vi "Write Tx Data (CDB WDT).vi"(0 "Register Bus":T1, 5 "data":waveform(cdb), 9 "timeout (s)":dbl=10.0, 11 "error in":errorcluster) -> (4 "Register Bus (out)":T1, 15 "error out":errorcluster)   [LabVIEW 2017]
doc: "Write Tx data to the device. It's required to call <b>Configure Stream</b> and <b>Initiate Stream</b> before calling this VI.\n\n<B>Input Parameters</B>\n\n<B>Register Bus</B> The Register Bus object created by the ni579x Open VI and used as the session handle for the NI-579x Configuration Design Library.\n\n<B>data</B> is the Tx data to write to the device.\n\n<B>timeout (s)</B> is how long to wait for (in seconds).\n\n<B>error in</B> describes error conditions that occur before this node runs. This input provides standard 'error in' functionality.\n\n<B>Output Parameters</B>\n\n<B>Register Bus (out)</B> The Register Bus object created by the ni579x Open VI and used as the session handle for the NI-579x Configuration Design Library.\n\n<B>error out</B> contains error information. This output provides standard 'error out' functionality."
uses:
  <instrlib>/_niInstr/Register Bus/v0/Host/Public/Register Bus Session.ctl
  <instrlib>/_niInstr/Register Bus/v0/Host/Private/Session Data.ctl
  Tx FPGA VI Reference.ctl
  <vilib>/Utility/error.llb/Error Cluster From Error Code.vi
  <vilib>/rvi/errors/niLvFpgaAdjustHostInterfaceError.vi
  <vilib>/rvi/interface/nirviMethod/nirviMethod.xnode
  <instrlib>/_niInstr/Register Bus/v0/Host/niInstr Register Bus v0 Host.lvlib
  <vilib>/FPGAPlugInAG/Dynamic/niLvFpga_WriteFifo_Dynamic.vi
  <vilib>/rvi/errors/niLvFpgaMergeErrorWithErrorCode.vi
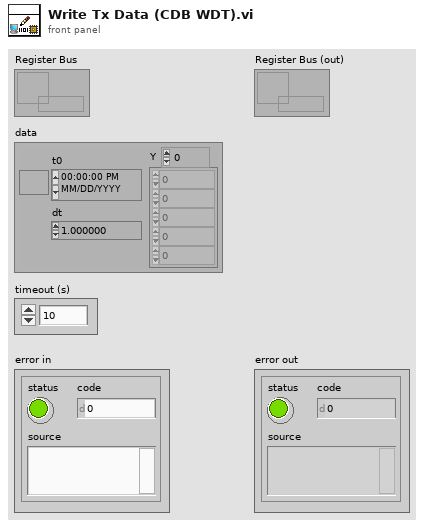
[diagram p1: front panel]
types:
  T1 = typedef "niInstr Register Bus v0 Host.lvlib/Register Bus Session.ctl" = refnum<queue>
  T2 = typedef "Tx FPGA VI Reference.ctl" = refnum<k20>
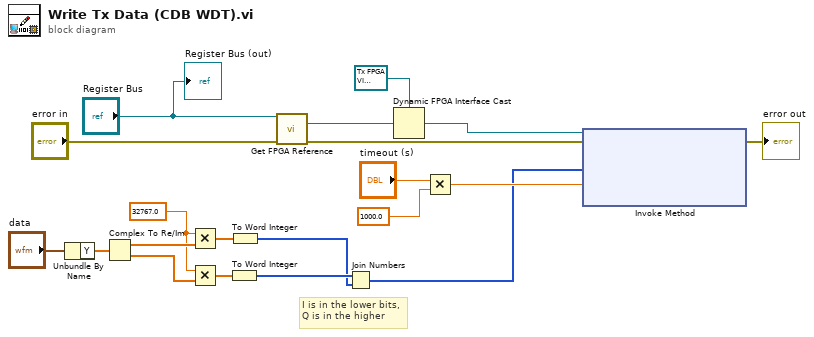
[diagram p0: block diagram]
diagram:
  w5 = 32767.0
  # "I is in the lower bits,\nQ is in the higher"
  n1 = Unbundle By Name("data") -> ("Y"=w8:cdb[])
  n2 = Complex To Re/Im(x + iy=w8) -> (x=w7:dbl[], y=w6:dbl[])
  n3 = Multiply(x=w5, y=w7) -> (x*y=w4:dbl[])
  n4 = Multiply(x=w5, y=w6) -> (x*y=w3:dbl[])
  n5 = To Word Integer(number=w3) -> (16bit integer=w2:i16[])
  n6 = To Word Integer(number=w4) -> (16bit integer=w1:i16[])
  n7 = call <instrlib>:"Get FPGA Reference.vi"("session in"="Register Bus", "error in"="error in") -> ("fpga ref"=w17:refnum<k20>, "error out"=w11:errorcluster)  [unwired: 11 in, 1 out]
  n8 = Join Numbers(hi=w2, lo=w1) -> ((hi.lo)=w10:u32[])
  n9 = Dynamic FPGA Interface Cast(Session In=T2 refnum ("Type"), Type=w17) -> (Session Out=w12:T2)
  n10 = Multiply(x="timeout (s)", y=1000.0) -> (x*y=w13:dbl)
  n11 = xnode "Invoke Method"("FPGA VI Reference In"=w12, "error in"=w11, "Data"=w10, "Timeout (ms)"=w13) -> ("error out"=→"error out":errorcluster)  [unwired: 2 out]
  "Register Bus (out)" <- "Register Bus"
